vi "Main.vi"() -> ()   [LabVIEW 2024]
uses:
  Consumer Message.ctl
  <vilib>/Utility/file.llb/Write Delimited Spreadsheet (DBL).vi
panel:
  out "Histogram":cluster{"histogram":dbl[], "x axis":dbl[]}(graph)
  in  "bins":i32=20
  in  "signal":u16(ring) items=["uniform white", "uniform+uniform", "Gaussian white", "sine", "square"]
  out "Consumer Shutdown?":bool
  out "Backlog":u8(slide) scale=0.0..100.0
  in  "Snapshot":bool
  in  "Stop":bool
  # "Number of enqueued messages waiting to be processed"
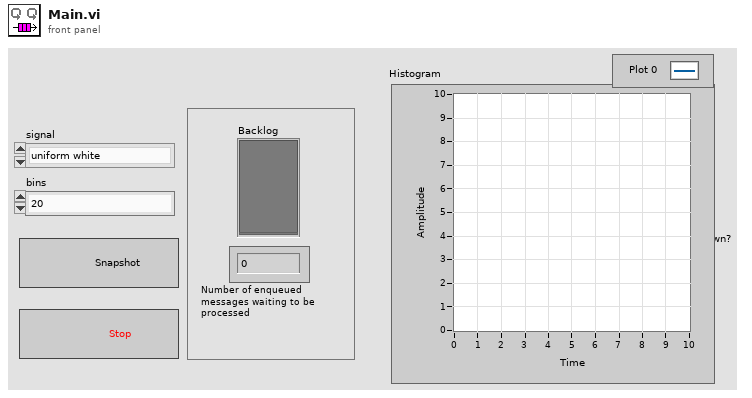
[diagram p1: front panel]
types:
  T1 = typedef "Consumer Message.ctl" = cluster{"Consumer State":string, "Boolean Data":bool, "Numeric Data":i32, "Signal":dbl[], "Error":errorcluster}
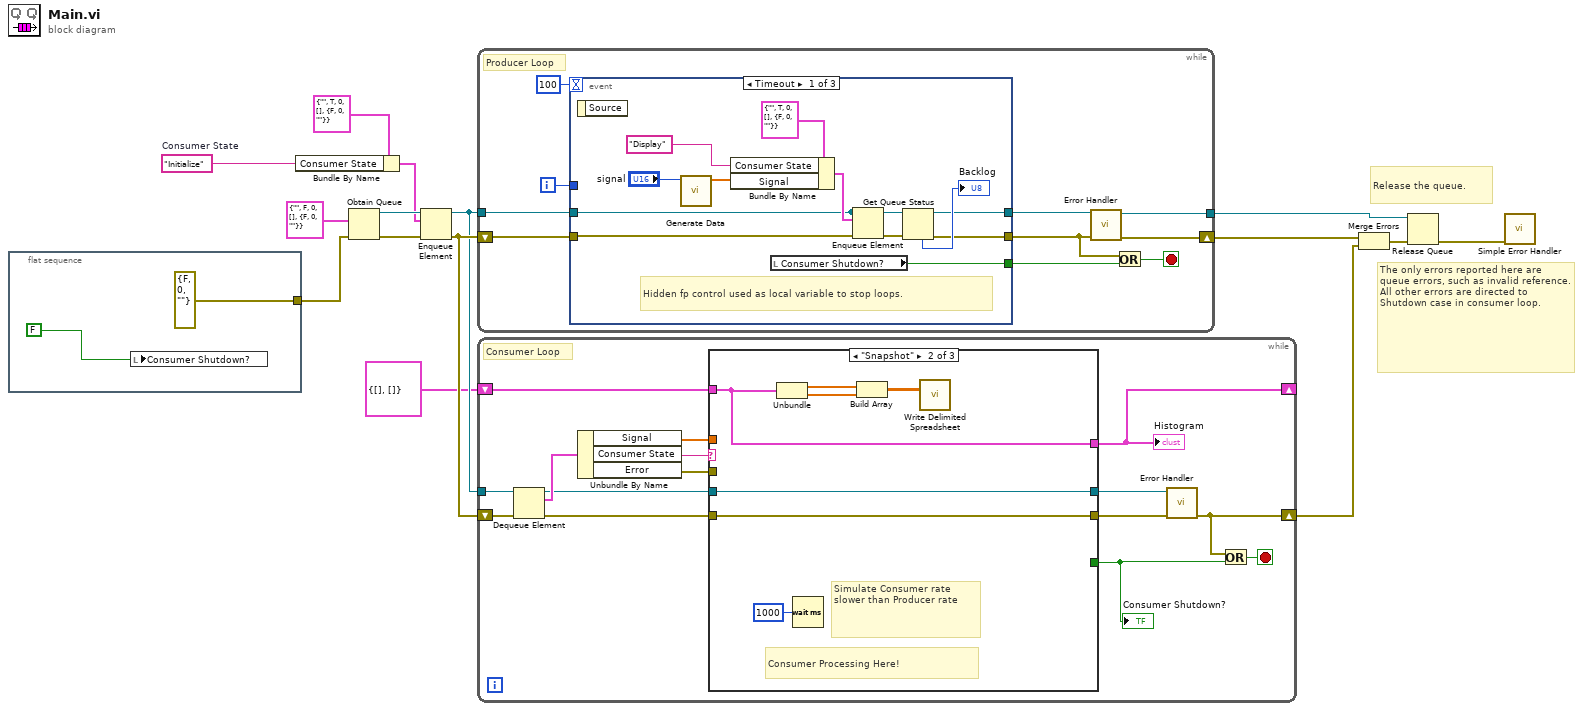
[diagram p0: block diagram]
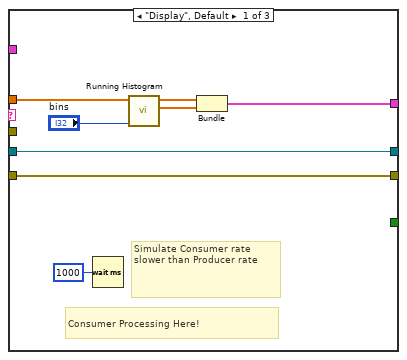
[diagram p2: hidden frame]
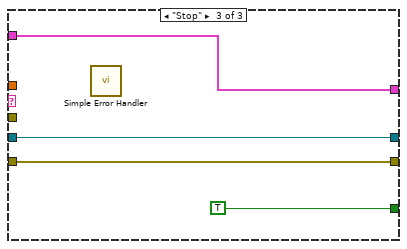
[diagram p3: hidden frame]
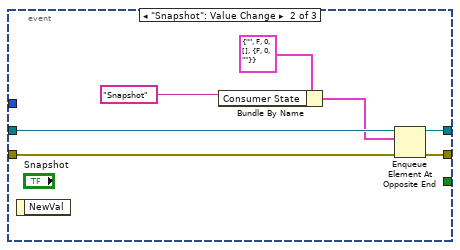
[diagram p4: hidden frame]
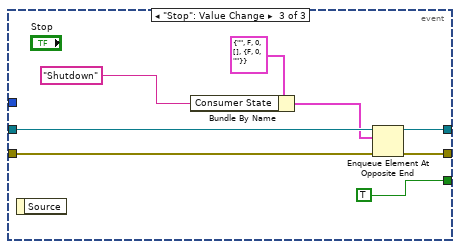
[diagram p5: hidden frame]
diagram:
  w7 = "Initialize"  # Consumer State
  # "Release the queue."
  # "The only errors reported here are queue errors, such as invalid reference.  All other errors are directed to Shutdown case in consumer loop."
  n1 = flat-sequence {
    tunnel: [errorcluster {"status"=FALSE, "code"=0, "source"=""} ("error in (no error)")] -> w10
    frame #0 {
      n2 = local write "Consumer Shutdown?"(FALSE ("Stop Loops (local)")) -> ()
    }
  }
  n3 = Bundle By Name(cluster=T1 {"Consumer State"="", "Boolean Data"=TRUE, "Numeric Data"=0, "Signal"=[], "Error"={"status"=FALSE, "code"=0, "source"=""}} ("Consumer Message"), "Consumer State"=w7) -> (w8:T1)
  n4 = Obtain Queue(element data type=T1 {"Consumer State"="", "Boolean Data"=FALSE, "Numeric Data"=0, "Signal"=[], "Error"={"status"=FALSE, "code"=0, "source"=""}}, error in (no error)=w10) -> (queue out=w12:refnum<queue>, error out=w15:errorcluster)  [unwired: 3 in, 1 out]
  n5 = Enqueue Element(queue=w12, element=w8, error in (no error)=w15) -> (queue out=w11:refnum<queue>, error out=w13:errorcluster)  [unwired: 1 in, 1 out]
  n6 = while {
    tunnel: w11 -> [w27]
    shift-right: [w19] -> w6
    shift-left: w13 -> [w26]
    tunnel: [w18] -> w2
    i -> [w25]
    stop <- w21 stop-if-true
    # "Producer Loop"
    n7 = event shown="[0] Timeout" {
      selector: _ -> [_ _ _]
      dyn-events: _ -> [_ _ _]
      timeout: 100 -> [_ _ _]
      tunnel: w27 -> [w28 w45 w54]
      tunnel: w26 -> [w30 w44 w52]
      tunnel: [w37 w46 w51] -> w20
      tunnel: [w39 _ TRUE] -> w22
      tunnel: w25 -> [_ _ _]
      tunnel: [w36 w41 w50] -> w24
      event Timeout {
        # "Hidden fp control used as local variable to stop loops."
        n8 = event-data() -> ()  [unwired: 1 in, 1 out]
        n9 = call "Generate Data.vi"("signal"="signal") -> ("Signal"=w34:dbl[])  [unwired: 9 in, 1 out]
        n10 = Bundle By Name(cluster=T1 {"Consumer State"="", "Boolean Data"=TRUE, "Numeric Data"=0, "Signal"=[], "Error"={"status"=FALSE, "code"=0, "source"=""}} ("Consumer Message"), "Consumer State"="Display", "Signal"=w34) -> (w31:T1)
        n11 = local read "Consumer Shutdown?"() -> (w39:bool)
        n12 = Enqueue Element(queue=w28, element=w31, error in (no error)=w30) -> (error out=w29:errorcluster)  [unwired: 1 in, 2 out]
        n13 = Get Queue Status(queue=w28, error in (no error)=w29) -> (queue out=w36:refnum<queue>, error out=w37:errorcluster, # elements in queue=→"Backlog":i32)  [unwired: 1 in, 5 out]
      }
      event "Snapshot": Value Change {
        n14 = event-data() -> ()  [unwired: 1 in, 1 out]
        n15 = Bundle By Name(cluster=T1 {"Consumer State"="", "Boolean Data"=FALSE, "Numeric Data"=0, "Signal"=[], "Error"={"status"=FALSE, "code"=0, "source"=""}}, "Consumer State"="Snapshot" ("String Data")) -> (w42:T1)
        n16 = Enqueue Element At Opposite End(queue=w45, element=w42, error in (no error)=w44) -> (queue out=w41:refnum<queue>, error out=w46:errorcluster)  [unwired: 1 in, 1 out]
      }
      event "Stop": Value Change {
        n17 = event-data() -> ()  [unwired: 1 in, 1 out]
        n18 = Bundle By Name(cluster=T1 {"Consumer State"="", "Boolean Data"=FALSE, "Numeric Data"=0, "Signal"=[], "Error"={"status"=FALSE, "code"=0, "source"=""}}, "Consumer State"="Shutdown") -> (w47:T1)
        n19 = Enqueue Element At Opposite End(queue=w54, element=w47, error in (no error)=w52) -> (queue out=w50:refnum<queue>, error out=w51:errorcluster)  [unwired: 1 in, 1 out]
      }
    }
    n20 = call "Error Handler.vi"("error in"=w20, "queue in"=w24) -> ("error out"=w19:errorcluster, "queue out"=w18:refnum<queue>)  [unwired: 8 in]
    n21 = Or(x=w20, y=w22) -> (x .or. y?=w21:bool)
  }
  n22 = while {
    tunnel: w11 -> [w69]
    shift-right: [w62] -> w5
    shift-left: w13 -> [w68]
    shift-right: [w56] -> _
    shift-left: cluster{"histogram":dbl[], "x axis":dbl[]} {"histogram"=[], "x axis"=[]} -> [w55]
    stop <- w63 stop-if-true
    # "Consumer Loop"
    n23 = Dequeue Element(queue=w69, error in (no error)=w68) -> (queue out=w61:refnum<queue>, element=w67:T1, error out=w60:errorcluster)  [unwired: 1 in, 1 out]
    n24 = Unbundle By Name(w67) -> ("Signal"=w57:dbl[], "Consumer State"=w58:string, "Error"=w59:errorcluster)
    n25 = case shown="\"Snapshot\"" w58 {
      tunnel: [_ _ TRUE] -> w64
      tunnel: w60 -> [w75 w82 w86]
      tunnel: [w75 w82 w86] -> w66
      tunnel: w61 -> [w77 w84 w87]
      tunnel: [w77 w84 w87] -> w65
      tunnel: w59 -> [_ _ _]
      tunnel: w57 -> [w74 _ _]
      tunnel: [w71 w78 w85] -> w56
      tunnel: w55 -> [_ w78 w85]
      frame "Display", Default {
        # "Simulate Consumer rate slower than Producer rate"
        # "Consumer Processing Here!"
        n26 = Wait (ms)(milliseconds to wait=u32 1000) -> ()  [unwired: 1 out]
        n27 = call "Running Histogram.vi"("bins"="bins", "input data"=w74) -> ("x axis"=w72:dbl[], "histogram"=w73:dbl[])  [unwired: 6 in, 2 out]
        n28 = Bundle("histogram"=w73, "x axis"=w72) -> (w71:cluster{"histogram":dbl[], "x axis":dbl[]})  [unwired: 1 in]
      }
      frame "Snapshot" {
        # "Simulate Consumer rate slower than Producer rate"
        # "Consumer Processing Here!"
        n29 = Unbundle "Unbundle"(w78) -> ("histogram"=w81:dbl[], "x axis"=w80:dbl[])
        n30 = Wait (ms)(milliseconds to wait=u32 1000) -> ()  [unwired: 1 out]
        n31 = Build Array "Build Array"(w81, w80) -> (w79:dbl[][])
        n32 = call-poly <vilib>:"Write Delimited Spreadsheet.vi"("2D data"=w79) -> ()  [unwired: 13 in, 2 out]
      }
      frame "Stop" {
        n33 = call <vilib>:"Simple Error Handler.vi"() -> ()  [unwired: 5 in, 5 out]
      }
    }
    "Consumer Shutdown?" <- w64
    "Histogram" <- w56
    n34 = call "Error Handler.vi"("error in"=w66, "queue in"=w65) -> ("error out"=w62:errorcluster)  [unwired: 8 in, 1 out]
    n35 = Or(x=w62, y=w64) -> (x .or. y?=w63:bool)
  }
  n36 = Merge Errors(w6, w5) -> (w4:errorcluster)
  n37 = Release Queue(queue=w2, error in (no error)=w4) -> (error out=w3:errorcluster)  [unwired: 1 in, 2 out]
  n38 = call <vilib>:"Simple Error Handler.vi"("error in (no error)"=w3) -> ()  [unwired: 4 in, 5 out]
